vi "Cable2MotorMismatch.vi"(3 "MotorTension":dbl[](array[numeric])) -> (0 "CableTension":dbl[](array[numeric]))   [LabVIEW 2015]
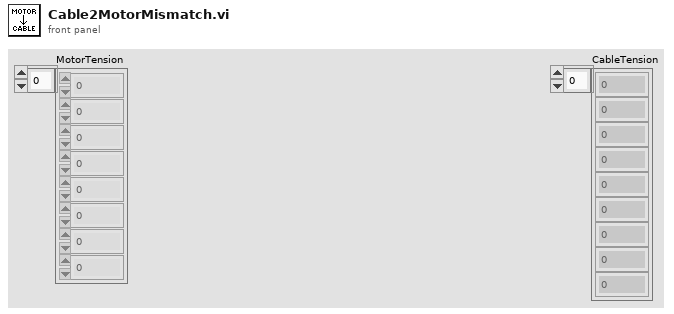
[diagram p1: front panel]
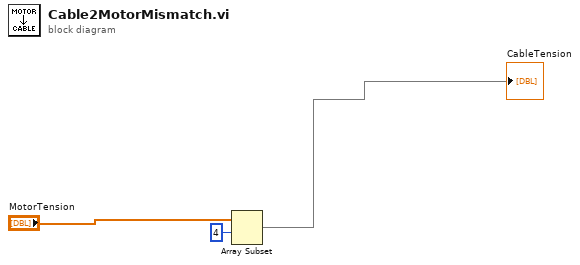
[diagram p0: block diagram]
diagram:
  n1 = Array Subset(array="MotorTension", index=4) -> (→"CableTension":dbl[])  [unwired: 1 in]
